vi "Read Power Measurement List Mode.vi"(6 "Step Index (1)":i32=1, 7 "Detector Type (RMS)":i32(ring) items=["RMS", "Minimum", "Maximum"], 8 "error in (no error)":errorcluster, 9 "Result Type (Current)":i32(ring) items=["Current", "Average", "Peak"], 10 "Instance (1)":i32=1, 11 "VISA resource name":refnum<visa-resource-name>) -> (0 "error out":errorcluster, 1 "Power":dbl format="%^.3e", 2 "Reliability":i32, 3 "VISA resource name out":refnum<visa-resource-name>)   [LabVIEW 2020, in "Rohde&Schwarz CMXP GPRF.lvlib"]
doc: "Starts ands returns the results of the GPRF power measurement for single step and \"Statistic\" evaluation mode.\n\nAttribute:\n-\n\nRemote-control commands:\nREAD:GPRF:MEAS<i>:POWer:LIST:CURRent?\nREAD:GPRF:MEAS<i>:POWer:LIST:MAXimum:CURRent?\nREAD:GPRF:MEAS<i>:POWer:LIST:MINimum:CURRent?\nREAD:GPRF:MEAS<i>:POWer:LIST:AVERage?\nREAD:GPRF:MEAS<i>:POWer:LIST:PEAK:MAXimum?\nREAD:GPRF:MEAS<i>:POWer:LIST:PEAK:MINimum?"
uses:
  <instrlib>/Rohde&Schwarz CMXP GPRF/Rohde&Schwarz CMXP GPRF.lvlib
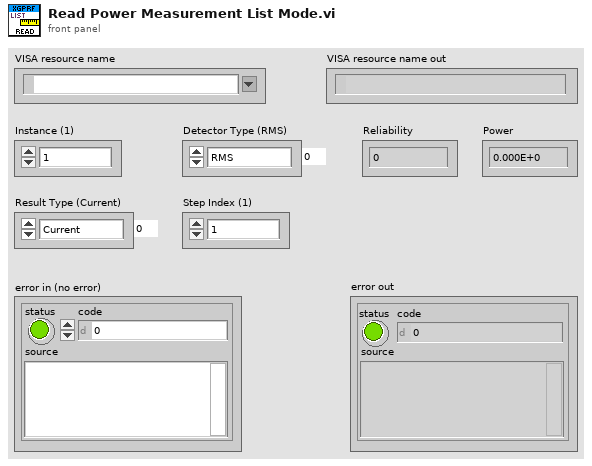
[diagram p1: front panel]
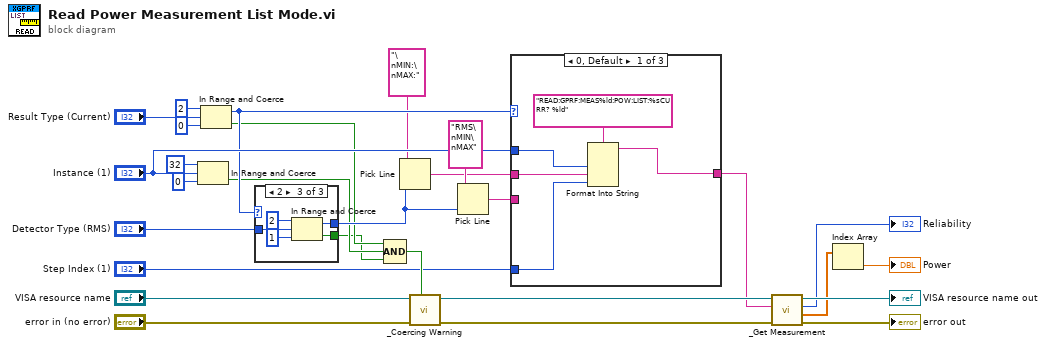
[diagram p0: block diagram]
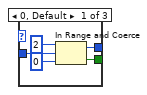
[diagram p2: hidden frame]
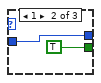
[diagram p3: hidden frame]
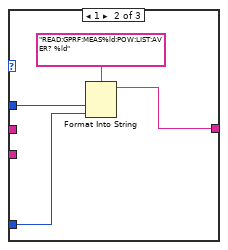
[diagram p4: hidden frame]
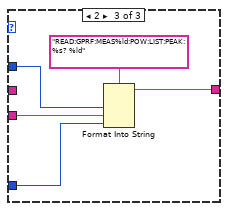
[diagram p5: hidden frame]
diagram:
  n1 = In Range and Coerce(upper limit=32, x="Instance (1)", lower limit=0) -> (In Range?=w4:bool)  [unwired: 1 out]
  n2 = In Range and Coerce(upper limit=2, x="Result Type (Current)", lower limit=0) -> (coerced(x)=w13:i32, In Range?=w3:bool)
  n3 = case shown="2" w13 {
    tunnel: [w31 TRUE w38] -> w1
    tunnel: [w30 w34 w37] -> w8
    tunnel: "Detector Type (RMS)" -> [w29 w34 w36]
    frame 0, Default {
      n4 = In Range and Coerce(upper limit=2, x=w29, lower limit=0) -> (coerced(x)=w30:i32, In Range?=w31:bool)
    }
    frame 1 {
    }
    frame 2 {
      n5 = In Range and Coerce(upper limit=2, x=w36, lower limit=1) -> (coerced(x)=w37:i32, In Range?=w38:bool)
    }
  }
  n6 = Compound Arithmetic op=AND(w3, w4, w1) -> (w26:bool)
  n7 = Pick Line(multi-line string="\nMIN:\nMAX:", line index=w8) -> (output string=w7:string)  [unwired: 1 in]
  n8 = call <instrlib>:"_Coercing Warning.vi"("In Range?"=w26, "error in (no error)"="error in (no error)", "VISA resource name"="VISA resource name") -> ("error out"=w22:errorcluster, "VISA resource name out"=w23:refnum<visa-resource-name>)  [unwired: 7 in]
  n9 = Pick Line(multi-line string="RMS\nMIN\nMAX", line index=w8) -> (output string=w6:string)  [unwired: 1 in]
  n10 = case shown="0, Default" w13 {
    tunnel: "Instance (1)" -> [w42 w48 w51]
    tunnel: [w44 w47 w53] -> w2
    tunnel: "Step Index (1)" -> [w41 w46 w50]
    tunnel: w7 -> [w43 _ _]
    tunnel: w6 -> [_ _ w52]
    frame 0, Default {
      n11 = Format Into String(format string="READ:GPRF:MEAS%ld:POW:LIST:%sCURR? %ld", w42, w43, w41) -> (resulting string=w44:string)  [unwired: 2 in, 1 out]
    }
    frame 1 {
      n12 = Format Into String(format string="READ:GPRF:MEAS%ld:POW:LIST:AVER? %ld", w48, w46) -> (resulting string=w47:string)  [unwired: 2 in, 1 out]
    }
    frame 2 {
      n13 = Format Into String(format string="READ:GPRF:MEAS%ld:POW:LIST:PEAK:%s? %ld", w51, w52, w50) -> (resulting string=w53:string)  [unwired: 2 in, 1 out]
    }
  }
  n14 = call <instrlib>:"_Get Measurement.vi"("error in (no error)"=w22, "Command"=w2, "VISA resource name"=w23) -> ("error out"=→"error out":errorcluster, "Data"=w11:dbl[], "Reliability"=→"Reliability":i32, "VISA resource name out"=→"VISA resource name out":refnum<visa-resource-name>)  [unwired: 5 in]
  n15 = Index Array(array=w11) -> (element=→"Power":dbl)  [unwired: 1 in]
